vi "fft_freq.vi"   [LabVIEW 2020]
uses:
  <vilib>/ptbypt/NI_PtbyPt.lvlib
  <vilib>/ptbypt/Frequency Domain.llb/Real FFT PtByPt.vi
  <vilib>/rvi/Analysis/host/Public/NI_FpgaMspHost.lvlib
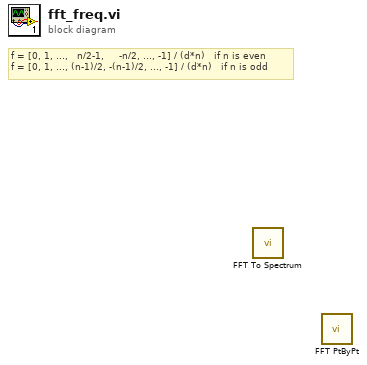
[diagram p0: block diagram]
diagram:
  # "f = [0, 1, ...,   n/2-1,     -n/2, ..., -1] / (d*n)   if n is even\nf = [0, 1, ..., (n-1)/2, -(n-1)/2, ..., -1] / (d*n)   if n is odd"
  n1 = call <vilib>:"FFT To Spectrum.vi"() -> ()  [unwired: 13 in, 3 out]
  n2 = call-poly <vilib>:"FFT PtByPt.vi"() -> ()  [unwired: 4 in, 2 out]
